vi "Global DAQ end.vi"() -> ()   [LabVIEW 2020]
panel:
  out "DAQ End Global":bool
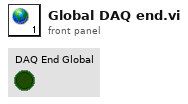
[diagram p1: front panel]
diagram:
